vi "数据查询_仪器日志.vi"() -> ()   [LabVIEW 2016, in "数据查询.lvlib"]
uses:
  <vilib>/Utility/miscctls.llb/LVPointTypeDef.ctl
  <vilib>/Utility/miscctls.llb/LVRowAndColumnUnsignedTypeDef.ctl
  <userlib>/_OpenG.lib/array/array.llb/Sort 2D Array (String)__ogtk.vi
  <userlib>/_LVST/sqlite_api/Core/Tables/SQLite_List Columns.vi
  <vilib>/addons/database/_DB Variant To Data/Database Variant To Data.xnode
panel:
  out "布尔":bool=TRUE
  in  "列表框":i32(listbox)
  in  "页":i32 format="第%.0f页"
  in  "每页条数":i32=1000
  in  "向后按钮":bool
  in  "向前按钮":bool
  in  "导出":bool
  in  "查询":bool
  out "数据表":string[][](table)
  in  "结束日期":string="2050/01/01"
  in  "起始日期":string="2010/01/01"
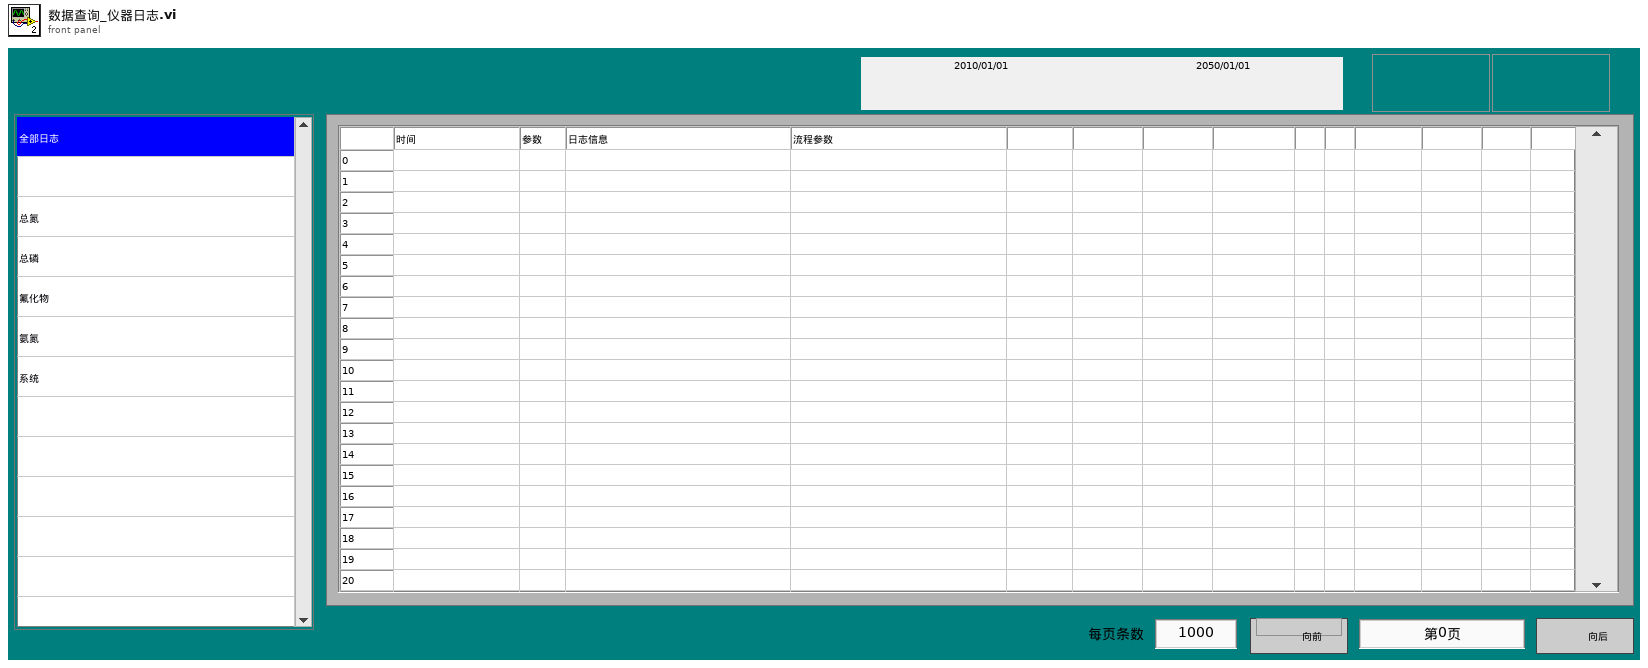
[diagram p1: front panel]
types:
  T1 = typedef "LVPointTypeDef.ctl" = cluster{"Horizontal":i16, "Vertical":i16}
  T2 = typedef "LVDateTimeRec.ctl" = cluster{"秒数的小数部分":dbl, "秒":i32, "分":i32, "时":i32, "日":i32, "月":i32, "年":i32, "天数（周）":i32, "天数（年）":i32, "DST":i32}
  T3 = typedef "Rendezvous RefNum" = refnum<k1>
  T4 = typedef "数据查询.lvlib/数据查询单选控件.ctl" = enum32{"数据查询", "仪器数据", "仪器日志", "报警信息", "校准日志"}
  T5 = typedef "数据库类型.ctl" = enum16{"Access", "SQLite"}
  T6 = enum8{"Enabled", "Disabled", "Disabled and Grayed Out"}
  T7 = typedef "LVRowAndColumnUnsignedTypeDef.ctl" = cluster{"Row":u32, "Column":u32}
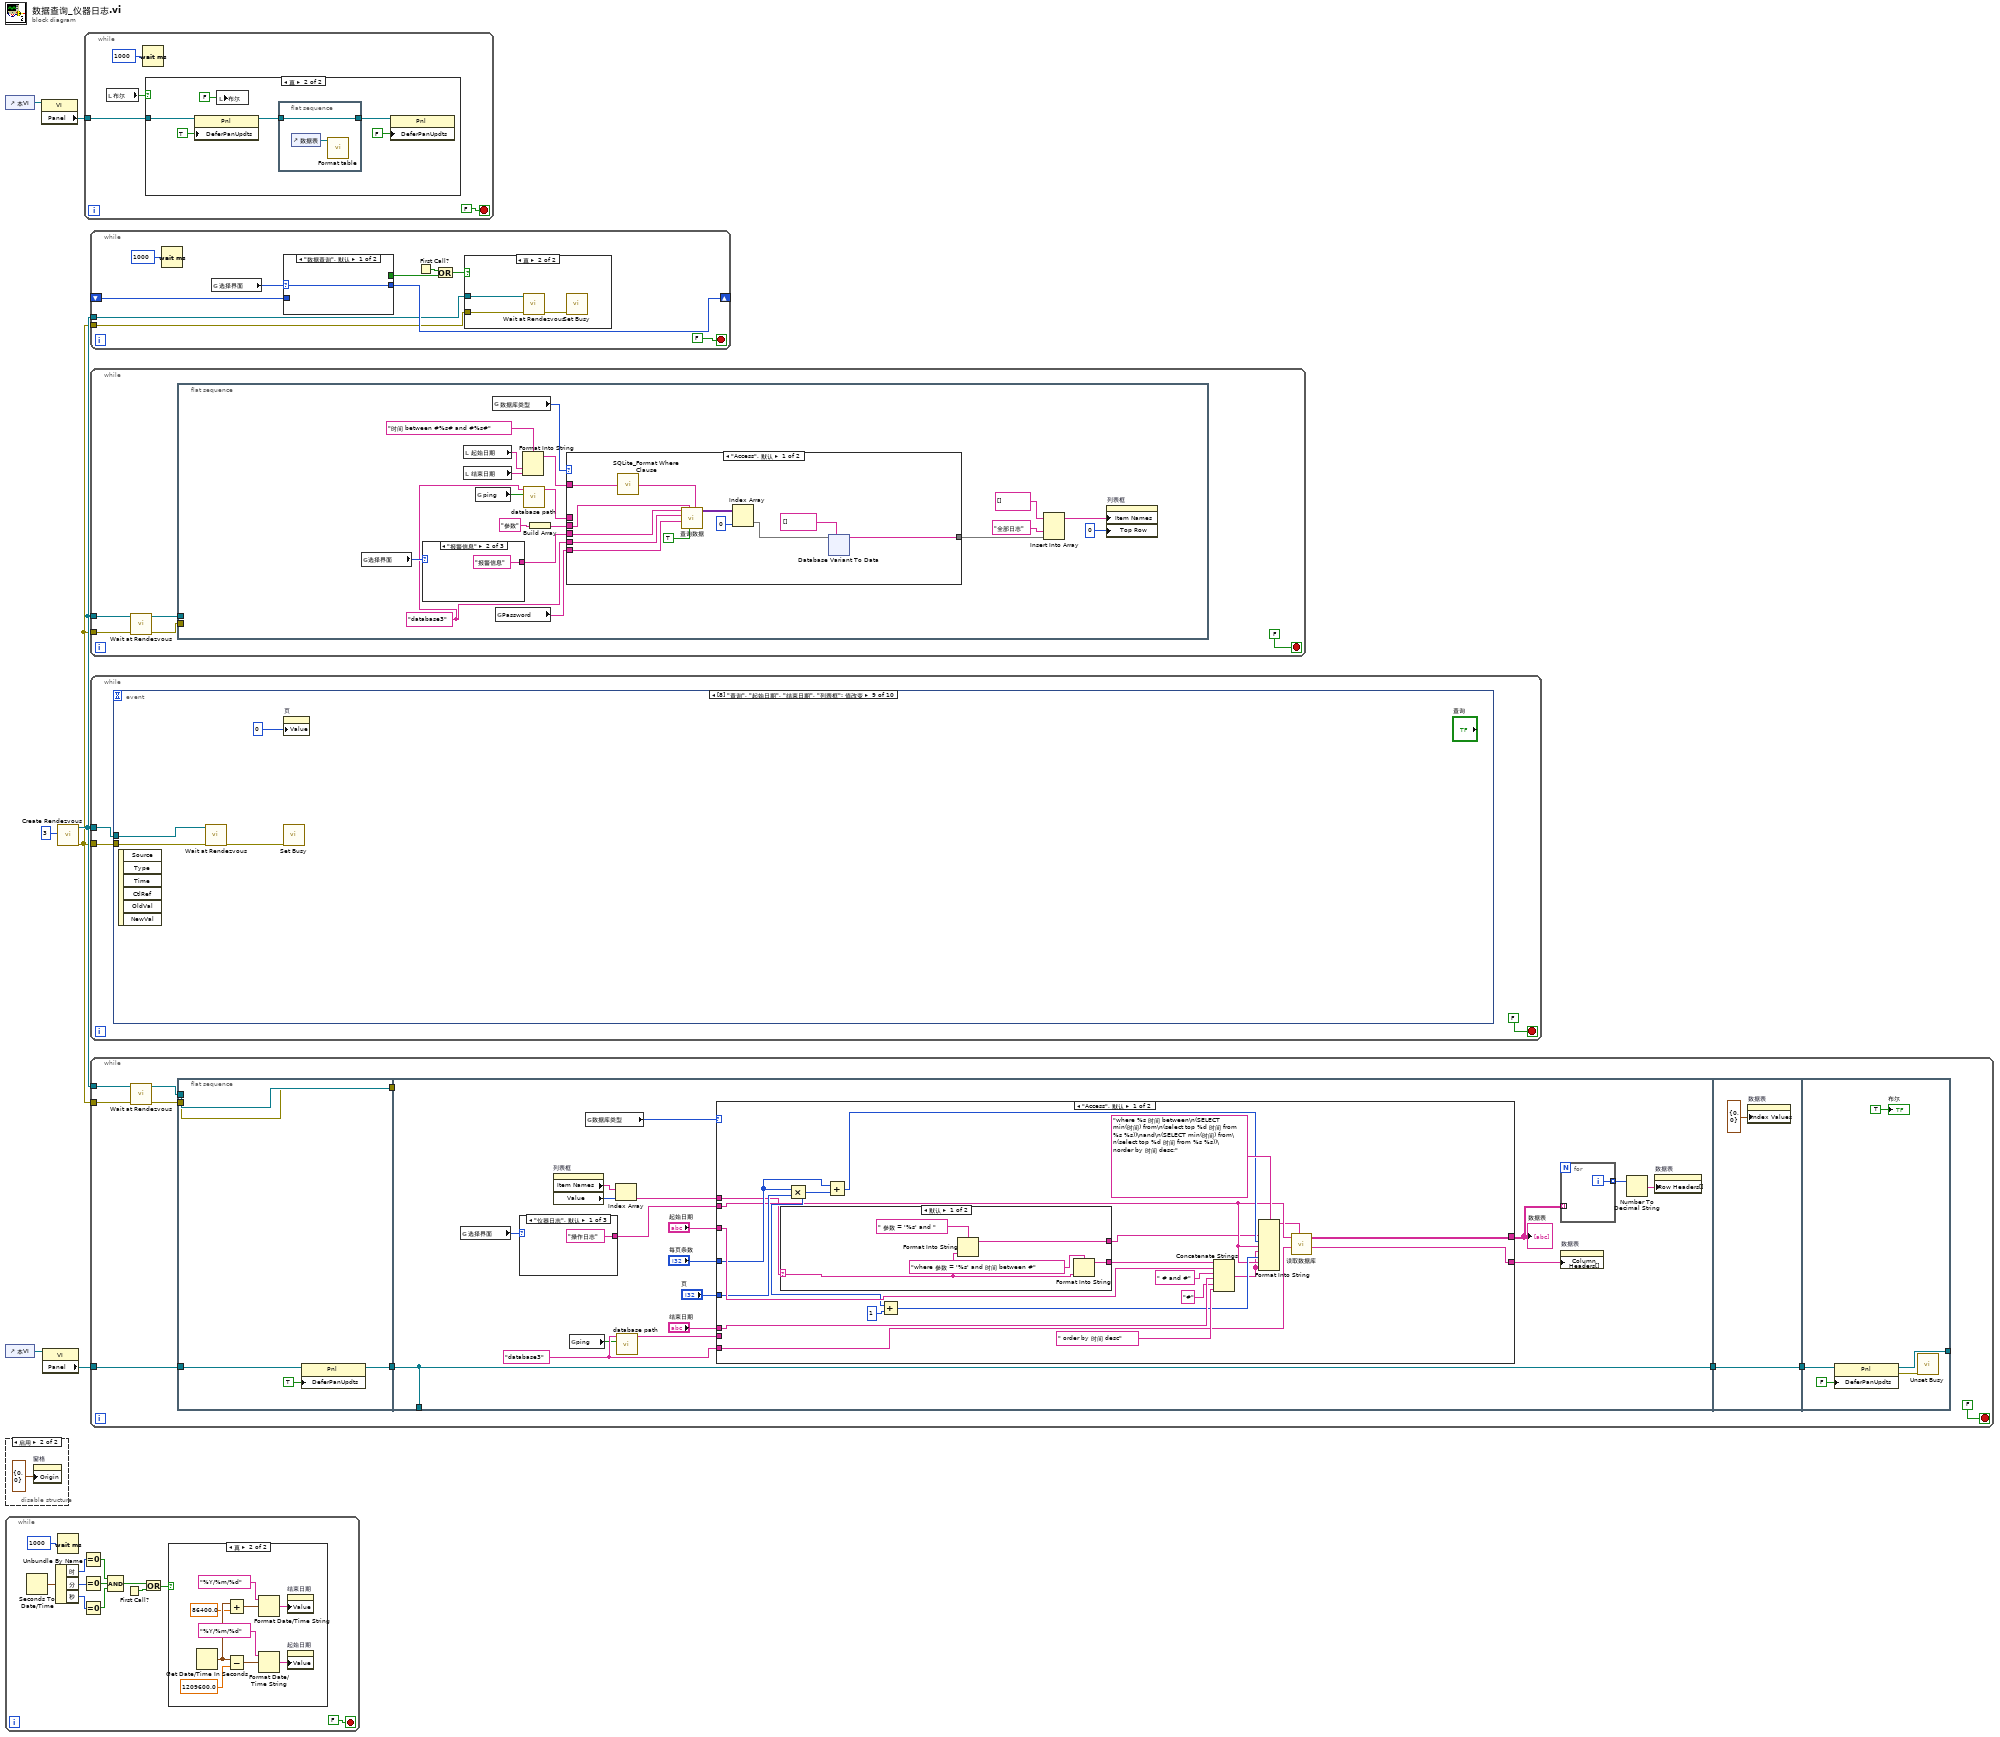
[diagram p0: block diagram]
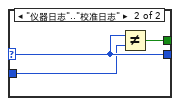
[diagram p4: hidden frame]
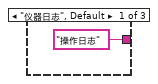
[diagram p5: hidden frame]
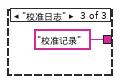
[diagram p6: hidden frame]
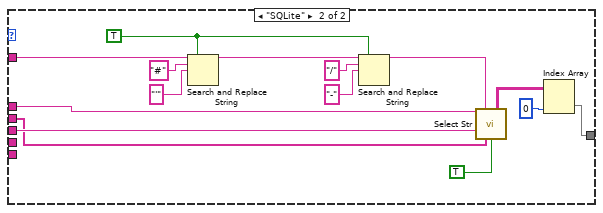
[diagram p7: hidden frame]
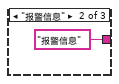
[diagram p8: hidden frame]
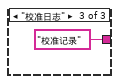
[diagram p9: hidden frame]
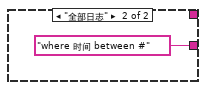
[diagram p10: hidden frame]
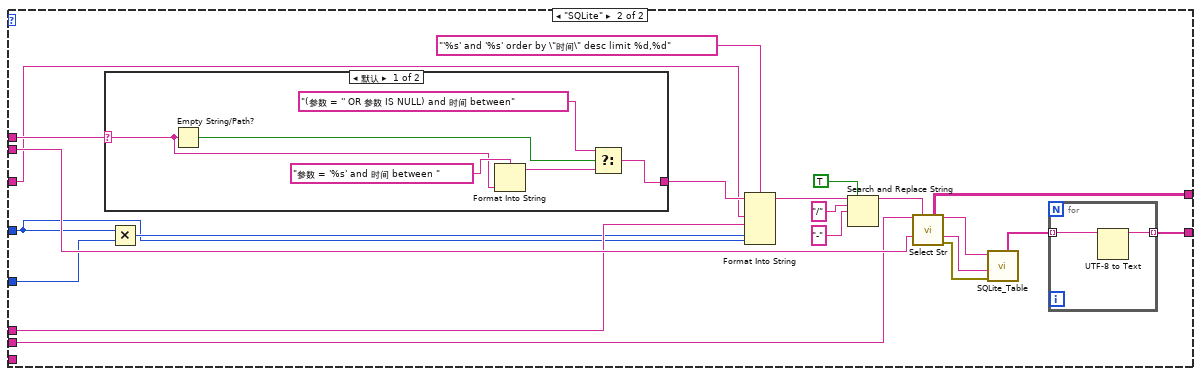
[diagram p11: hidden frame]
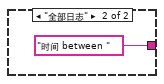
[diagram p12: hidden frame]
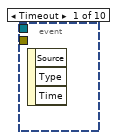
[diagram p14: hidden frame]
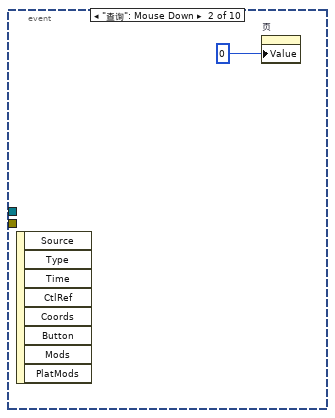
[diagram p15: hidden frame]
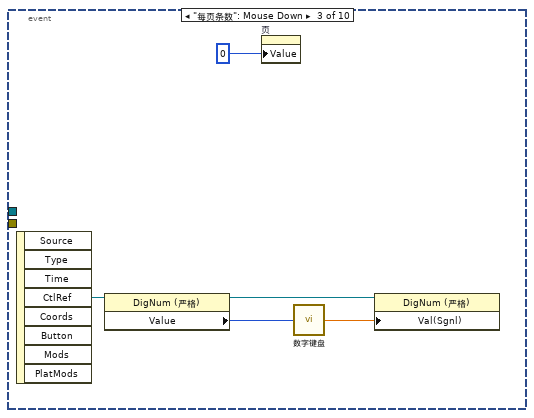
[diagram p16: hidden frame]
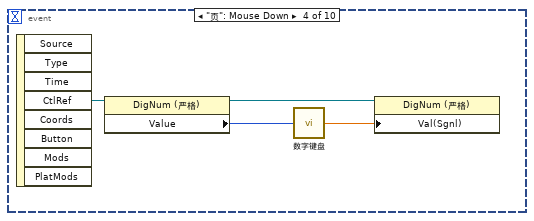
[diagram p17: hidden frame]
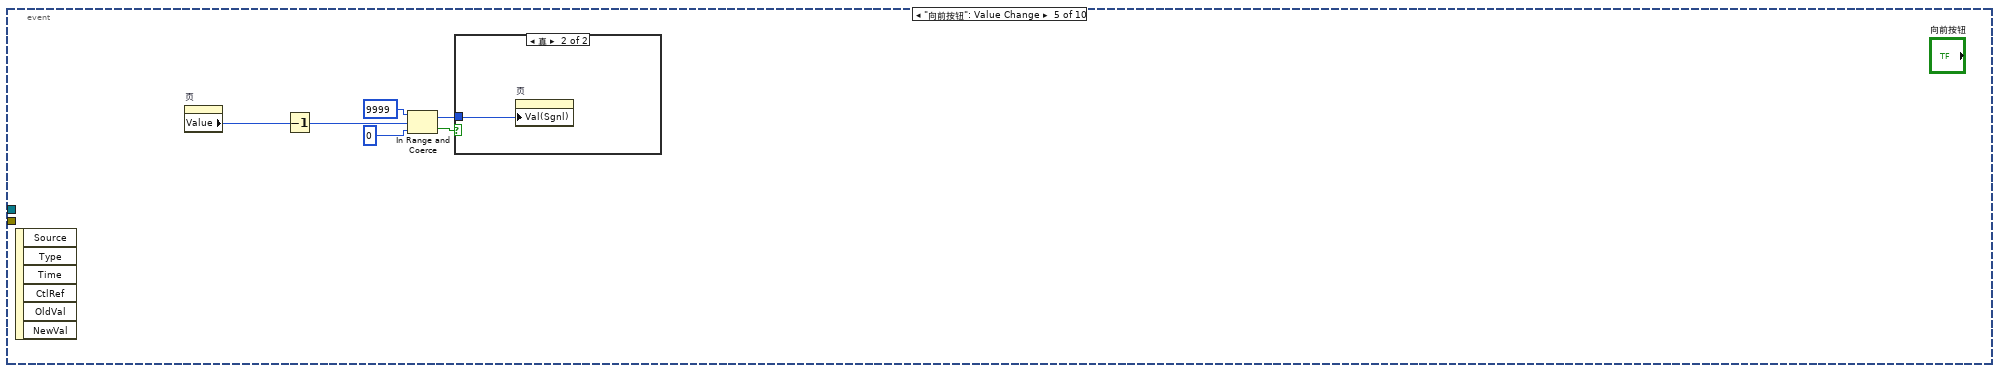
[diagram p18: hidden frame]
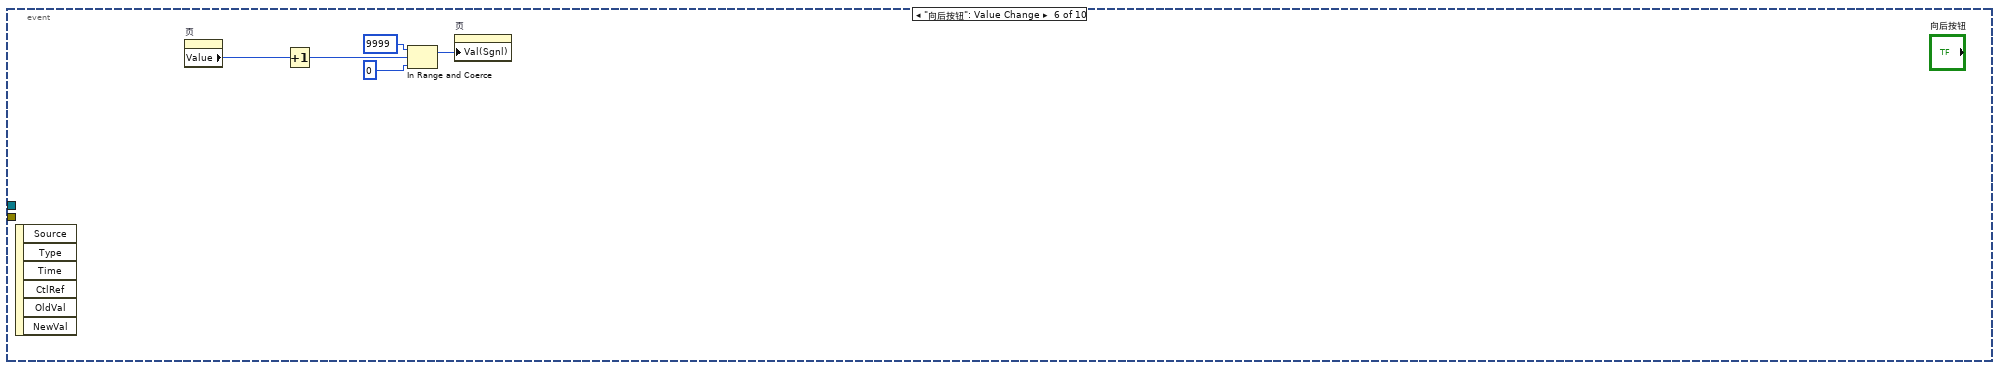
[diagram p20: hidden frame]
diagram:
  n1 = control-ref of="本VI"() -> (w2:refnum<vi>)
  n2 = control-ref of="本VI"() -> (w6:refnum<vi>)
  n3 = disable-structure shown="启用" {
    frame Disabled {
    }
    frame Enabled {
      n4 = property on="窗格" class="Pane"("Origin"=T1 {"Horizontal"=0, "Vertical"=0} ("原点")) -> ()  [unwired: 2 in, 2 out]
    }
  }
  n5 = while {
    stop <- FALSE stop-if-true
    n6 = Seconds To Date/Time() -> (date time rec=w20:T2)  [unwired: 2 in]
    n7 = Unbundle By Name(w20) -> ("时"=w19:i32, "分"=w18:i32, "秒"=w17:i32)
    n8 = Wait (ms)(milliseconds to wait=u32 1000 ("等待时间（毫秒）")) -> ()  [unwired: 1 out]
    n9 = Equal To 0?(x=w19) -> (x = 0?=w16:bool)
    n10 = Equal To 0?(x=w18) -> (x = 0?=w15:bool)
    n11 = Equal To 0?(x=w17) -> (x = 0?=w14:bool)
    n12 = Compound Arithmetic op=AND ("复合运算")(w16, w15, w14) -> (w11:bool)
    n13 = First Call?() -> (First Call?: T/F=w10:bool)
    n14 = Or(x=w11, y=w10) -> (x .or. y?=w9:bool)
    n15 = case shown="真" w9 {
      frame False {
      }
      frame True {
        n16 = Get Date/Time In Seconds() -> (seconds since 1Jan1904=w25:timestamp)
        n17 = Add(x=w25, y=86400.0) -> (x+y=w23:timestamp)
        n18 = Subtract(x=w25, y=1209600.0) -> (x-y=w26:timestamp)
        n19 = Format Date/Time String(time format string (%c)="%Y/%m/%d" ("时间格式字符串(%c)"), seconds (now)=w23) -> (date/time string=w22:string)  [unwired: 1 in]
        n20 = Format Date/Time String(time format string (%c)="%Y/%m/%d" ("时间格式字符串(%c)"), seconds (now)=w26) -> (date/time string=w28:string)  [unwired: 1 in]
        n21 = property on="结束日期" class="Str"("Value"=w22) -> ()  [unwired: 2 in, 2 out]
        n22 = property on="起始日期" class="Str"("Value"=w28) -> ()  [unwired: 2 in, 2 out]
      }
    }
  }
  n23 = property class="VI"(reference=w2) -> ("Panel"=w1:refnum<vi>)  [unwired: 1 in, 2 out]
  n24 = property class="VI"(reference=w6) -> ("Panel"=w5:refnum<vi>)  [unwired: 1 in, 2 out]
  n25 = call <vilib>:"Create Rendezvous.vi"("size (2)"=3) -> ("error out"=w3:errorcluster, "rendezvous"=w4:T3)  [unwired: 4 in, 1 out]
  n26 = while {
    tunnel: w1 -> [w32]
    stop <- FALSE stop-if-true
    n27 = local read "布尔"() -> (w31:bool)
    n28 = Wait (ms)(milliseconds to wait=u32 1000 ("等待时间（毫秒）")) -> ()  [unwired: 1 out]
    n29 = case shown="真" w31 {
      tunnel: w32 -> [_ w38]
      frame False {
      }
      frame True {
        n30 = property class="Pnl"(reference=w38, "DeferPanUpdts"=TRUE ("延迟前面板更新")) -> (reference out=w37:refnum<vi>)  [unwired: 1 in, 1 out]
        n31 = local write "布尔"(FALSE ("布尔")) -> ()
        n32 = flat-sequence {
          tunnel: [w40] -> w36
          tunnel: w37 -> [w40]
          frame #0 {
            n33 = control-ref of="数据表"() -> (w41:refnum<vi>)
            n34 = call "Format table.vi"("Table输入"=w41) -> ()  [unwired: 11 in]
          }
        }
        n35 = property class="Pnl"(reference=w36, "DeferPanUpdts"=FALSE ("延迟前面板更新")) -> ()  [unwired: 1 in, 2 out]
      }
    }
  }
  n36 = while {
    shift-right: [w48] -> _
    shift-left: _ -> [w47]
    tunnel: w4 -> [w45]
    tunnel: w3 -> [w42]
    stop <- FALSE stop-if-true
    n37 = Wait (ms)(milliseconds to wait=u32 1000 ("等待时间（毫秒）")) -> ()  [unwired: 1 out]
    n38 = global read "全局变量.vi" "选择界面"() -> (w49:T4)
    n39 = case shown="\"数据查询\", 默认" w49 {
      selector: w49 -> [w55 w58]
      tunnel: [w55 w58] -> w48
      tunnel: w47 -> [_ w57]
      tunnel: [_ w56] -> w46
      frame "数据查询", Default {
      }
      frame "仪器日志".."校准日志" {
        n40 = Not Equal?(x=w58, y=w57) -> (x != y?=w56:bool)
      }
    }
    n41 = First Call?() -> (First Call?: T/F=w43:bool)
    n42 = Or(x=w43, y=w46) -> (x .or. y?=w44:bool)
    n43 = case shown="真" w44 {
      tunnel: w45 -> [_ w54]
      tunnel: w42 -> [_ w53]
      frame False {
      }
      frame True {
        n44 = call <vilib>:"Wait at Rendezvous.vi"("error in (no error)"=w53, "rendezvous"=w54) -> ("error out"=w52:errorcluster)  [unwired: 3 in, 2 out]
        n45 = call <vilib>:"Set Busy.vi"("error in (no error)"=w52) -> ()  [unwired: 9 in, 2 out]
      }
    }
  }
  n46 = while {
    tunnel: w4 -> [w62]
    tunnel: w3 -> [w61]
    stop <- FALSE stop-if-true
    n47 = call <vilib>:"Wait at Rendezvous.vi"("error in (no error)"=w61, "rendezvous"=w62) -> ("error out"=w59:errorcluster, "rendezvous out"=w60:T3)  [unwired: 3 in, 1 out]
    n48 = flat-sequence {
      tunnel: w60 -> [_]
      tunnel: w59 -> [_]
      frame #0 {
        w68 = "database3" ("database")
        n49 = global read "全局变量.vi" "选择界面"() -> (w71:T4)
        n50 = case shown="\"报警信息\"" w71 {
          tunnel: ["操作日志" "报警信息" "校准记录"] -> w70
          frame "仪器日志", Default {
          }
          frame "报警信息" {
          }
          frame "校准日志" {
          }
        }
        n51 = local read "起始日期"() -> (w77:string)
        n52 = local read "结束日期"() -> (w76:string)
        n53 = global read "全局变量.vi" "ping"() -> (w67:bool)
        n54 = global read "外部调用接口全局变量.vi" "数据库类型"() -> (w65:T5)
        n55 = global read "外部调用接口全局变量.vi" "Password"() -> (w64:string)
        n56 = Format Into String(format string="时间 between #%s# and #%s#" ("格式字符串"), w77, w76) -> (resulting string=w73:string)  [unwired: 2 in, 1 out]
        n57 = call "database path.vi"("ping"=w67, "database"=w68) -> ("Path out"=w69:string)  [unwired: 8 in, 1 out]
        n58 = Build Array("参数") -> (w72:string[])
        n59 = case shown="\"Access\", 默认" w65 {
          tunnel: w70 -> [w96 w149]
          tunnel: w72 -> [w95 w148]
          tunnel: [w89 w135] -> w66
          tunnel: w73 -> [w88 w144]
          tunnel: w68 -> [w86 _]
          tunnel: w69 -> [_ w136]
          tunnel: w64 -> [w85 _]
          frame "Access", Default {
            n60 = call <userlib>:"SQLite_Format Where Clause.vi"("Where clause"=w88) -> ("String"=w87:string)  [unwired: 4 in]
            n61 = call "查询数据.vi"("condition"=w87, "Distinct"=TRUE, "columns"=w95, "Password"=w85, "database"=w86, "table"=w96) -> ("data"=w94:variant[][])  [unwired: 4 in, 1 out]
            n62 = Index Array(array=w94, index (col)=0 ("禁用的索引 (列)")) -> (element=w93:variant[])  [unwired: 1 in]
            n63 = xnode "Database Variant To Data"("database variant"=w93, "type"=string[] []) -> ("data"=w89:string[])  [unwired: 1 in, 1 out]
          }
          frame "SQLite" {
            w137 = TRUE ("替换全部？(F)")
            n64 = Search and Replace String(replace all?=w137, input string=w144, search string="#" ("搜索字符串"), replace string="'" ("替换字符串(\"\")")) -> (result string=w139:string)  [unwired: 4 in, 3 out]
            n65 = Search and Replace String(replace all?=w137, input string=w139, search string="/" ("搜索字符串"), replace string="-" ("替换字符串(\"\")")) -> (result string=w138:string)  [unwired: 4 in, 3 out]
            n66 = call "Select Str.vi"("DB Path"=w136, "Where Clause"=w138, "Tables Name"=w149, "Columns"=w148, "Distinct"=TRUE) -> ("Results"=w146:string[][])  [unwired: 7 in, 3 out]
            n67 = Index Array(array=w146, index (col)=0 ("禁用的索引 (列)")) -> (element=w135:string[])  [unwired: 1 in]
          }
        }
        n68 = Insert Into Array(array=string[] [], new element #1="全部日志" ("新元素/子数组"), new element #2=w66) -> (w75:string[])  [unwired: 1 in]
        n69 = property on="列表框" class="LstBox (严格)"("Item Names"=w75, "Top Row"=0 ("顶行")) -> ()  [unwired: 2 in, 2 out]
      }
    }
  }
  n70 = while {
    tunnel: w4 -> [w151]
    tunnel: w3 -> [w150]
    stop <- FALSE stop-if-true
    n71 = event shown="[8] \"查询\", \"起始日期\", \"结束日期\", \"列表框\": 值改变" {
      selector: _ -> [_ _ _ _ _ _ _ _ _ _]
      dyn-events: _ -> [_ _ _ _ _ _ _ _ _ _]
      timeout: _ -> [_ _ _ _ _ _ _ _ _ _]
      tunnel: w151 -> [_ _ _ _ _ _ _ _ w221 w225]
      tunnel: w150 -> [_ _ _ _ _ _ _ _ w220 w224]
      event Timeout {
        n72 = event-data() -> ()  [unwired: 1 in, 3 out]
      }
      event "查询": Mouse Down {
        n73 = event-data() -> ()  [unwired: 1 in, 8 out]
        n74 = property on="页" class="DigNum (严格)"("Value"=0 ("页")) -> ()  [unwired: 2 in, 2 out]
      }
      event "每页条数": Mouse Down {
        n75 = event-data() -> ("CtlRef"=w158:refnum<vi>)  [unwired: 1 in, 7 out]
        n76 = property class="DigNum (严格)"(reference=w158) -> (reference out=w155:refnum<vi>, "Value"=w157:i32)  [unwired: 1 in, 1 out]
        n77 = property on="页" class="DigNum (严格)"("Value"=0 ("页")) -> ()  [unwired: 2 in, 2 out]
        n78 = call "数字键盘.vi"("OldNumber"=w157) -> ("NewNumber"=w156:sgl)
        n79 = property class="DigNum (严格)"(reference=w155, "Val(Sgnl)"=w156) -> ()  [unwired: 1 in, 2 out]
      }
      event "页": Mouse Down {
        n80 = event-data() -> ("CtlRef"=w162:refnum<vi>)  [unwired: 1 in, 7 out]
        n81 = property class="DigNum (严格)"(reference=w162) -> (reference out=w159:refnum<vi>, "Value"=w161:i32)  [unwired: 1 in, 1 out]
        n82 = call "数字键盘.vi"("OldNumber"=w161) -> ("NewNumber"=w160:sgl)
        n83 = property class="DigNum (严格)"(reference=w159, "Val(Sgnl)"=w160) -> ()  [unwired: 1 in, 2 out]
      }
      event "向前按钮": Value Change {
        n84 = event-data() -> ()  [unwired: 1 in, 6 out]
        n85 = property on="页" class="DigNum (严格)"() -> ("Value"=w168:i32)  [unwired: 2 in, 2 out]
        n86 = Decrement(x=w168) -> (x-1=w167:i32)
        n87 = In Range and Coerce(upper limit=9999 ("上限"), x=w167, lower limit=0 ("下限")) -> (coerced(x)=w164:i32, In Range?=w163:bool)
        n88 = case shown="真" w163 {
          tunnel: w164 -> [_ w169]
          frame False {
          }
          frame True {
            n89 = property on="页" class="DigNum (严格)"("Val(Sgnl)"=w169) -> ()  [unwired: 2 in, 2 out]
          }
        }
      }
      event "向后按钮": Value Change {
        n90 = event-data() -> ()  [unwired: 1 in, 6 out]
        n91 = property on="页" class="DigNum (严格)"() -> ("Value"=w174:i32)  [unwired: 2 in, 2 out]
        n92 = Increment(x=w174) -> (x+1=w173:i32)
        n93 = In Range and Coerce(upper limit=u32 9999 ("上限"), x=w173, lower limit=u32 0 ("下限")) -> (coerced(x)=w170:u32)  [unwired: 1 out]
        n94 = property on="页" class="DigNum (严格)"("Val(Sgnl)"=w170) -> ()  [unwired: 2 in, 2 out]
      }
      event "导出": Value Change {
        n95 = event-data() -> ("CtlRef"=w175:refnum<vi>)  [unwired: 1 in, 5 out]
        n96 = property class="Bool"(reference=w175, "DisabledEnum"=T6."Disabled and Grayed Out" ("禁用")) -> (reference out=w179:refnum<vi>, error out=w180:errorcluster)  [unwired: 1 in]
        n97 = flat-sequence {
          tunnel: w180 -> [_]
          tunnel: [w199] -> w178
          tunnel: w179 -> [w199]
          tunnel: "导出" -> [_]
          frame #0 {
            n98 = local read "数据表"() -> (w203:string[][])
            n99 = call-poly <userlib>:"Sort Array__ogtk.vi"("Column/Row to Sort By"=u32 0, "Sort By in"=enum16{"row", "column"}."column", "Order"=enum16{"ascending", "descending"}."ascending", "Array in"=w203) -> ("Sorted Array out"=w185:string[][])  [unwired: 4 in, 3 out]
            n100 = for {
              tunnel: w185 -> [w212] mode=indexing
              tunnel: [w211] -> w189 mode=indexing
              i -> [w213]
              n101 = Increment(x=w213) -> (x+1=w209:i32)
              n102 = Number To Decimal String(number=w209) -> (decimal integer string=w208:string)  [unwired: 1 in]
              n103 = Insert Into Array(array=w212, index=0 ("索引"), new element=w208) -> (w211:string[])
            }
            n104 = property on="数据表" class="Tbl (严格)"() -> ("Column Headers[]"=w192:string[])  [unwired: 2 in, 2 out]
            n105 = property on="列表框" class="LstBox (严格)"() -> ("Item Names"=w184:string[], "Value"=w183:i32)  [unwired: 2 in, 2 out]
            n106 = Insert Into Array(array=w192, index=0 ("索引"), new element="序号" ("新元素/子数组")) -> (w193:string[])
            n107 = Index Array(array=w184, index=w183) -> (element=w182:string)
            n108 = Format Date/Time String(time format string (%c)="%y_%m_%d" ("时间格式字符串(%c)")) -> (date/time string=w196:string)  [unwired: 2 in]
            n109 = Concatenate Strings(w182, "_" ("字符串"), w196) -> (w194:string)
            n110 = Insert Into Array(array=string[][] [], new element #1=w193, new element #2=w189) -> (w188:string[][])  [unwired: 2 in]
            n111 = call "数据导出Excel.vi"("text data"=w188, "default name"=w194) -> ("error out"=w187:errorcluster, "布尔"=w186:bool)  [unwired: 8 in]
            n112 = case shown="真" w186 {
              tunnel: w187 -> [_ w205]
              frame False {
              }
              frame True {
                n113 = case shown="错误" w205 {
                  tunnel: ["导出成功" ("消息") "导出失败" ("消息")] -> w204
                  frame No Error {
                  }
                  frame Error {
                  }
                }
                n114 = One Button Dialog(message=w204) -> ()  [unwired: 1 in, 1 out]
              }
            }
          }
        }
        n115 = property class="Bool"(reference=w178, "DisabledEnum"=T6."Enabled" ("禁用")) -> ()  [unwired: 1 in, 2 out]
      }
      event "起始日期", "结束日期": Mouse Down {
        n116 = event-data() -> ("CtlRef"=w218:refnum<vi>)  [unwired: 1 in, 7 out]
        n117 = property class="Str"(reference=w218) -> (reference out=w216:refnum<vi>, "Value"=w217:string)  [unwired: 1 in, 1 out]
        n118 = property on="页" class="DigNum (严格)"("Value"=0 ("页")) -> ()  [unwired: 2 in, 2 out]
        n119 = call "日期键盘.vi"("原值"=w217) -> ("x+y"=w215:string)  [unwired: 10 in]
        n120 = property class="Str"(reference=w216, "Val(Sgnl)"=w215) -> ()  [unwired: 1 in, 2 out]
      }
      event "查询", "起始日期", "结束日期", "列表框": Value Change {
        n121 = event-data() -> ()  [unwired: 1 in, 6 out]
        n122 = call <vilib>:"Wait at Rendezvous.vi"("error in (no error)"=w220, "rendezvous"=w221) -> ("error out"=w219:errorcluster)  [unwired: 3 in, 2 out]
        n123 = property on="页" class="DigNum (严格)"("Value"=0 ("页")) -> ()  [unwired: 2 in, 2 out]
        n124 = call <vilib>:"Set Busy.vi"("error in (no error)"=w219) -> ()  [unwired: 9 in, 2 out]
      }
      event "页", "每页条数": Value Change {
        n125 = event-data() -> ()  [unwired: 1 in, 6 out]
        n126 = call <vilib>:"Wait at Rendezvous.vi"("error in (no error)"=w224, "rendezvous"=w225) -> ("error out"=w223:errorcluster)  [unwired: 3 in, 2 out]
        n127 = call <vilib>:"Set Busy.vi"("error in (no error)"=w223) -> ()  [unwired: 9 in, 2 out]
      }
    }
  }
  n128 = while {
    tunnel: w4 -> [w235]
    tunnel: w3 -> [w234]
    tunnel: w5 -> [w229]
    stop <- FALSE stop-if-true
    n129 = call <vilib>:"Wait at Rendezvous.vi"("error in (no error)"=w234, "rendezvous"=w235) -> ("error out"=w232:errorcluster, "rendezvous out"=w233:T3)  [unwired: 3 in, 1 out]
    n130 = flat-sequence {
      tunnel: w232 -> [w240]
      tunnel: w233 -> [w241]
      tunnel: [w241] -> w231
      tunnel: [w240] -> w230
      tunnel: w229 -> [w239]
      tunnel: [w237] -> w228
      tunnel: w231 -> [_]
      tunnel: w230 -> [_]
      tunnel: [w242] -> _
      tunnel: w228 -> [w242]
      tunnel: [w242] -> w227
      tunnel: w227 -> [w321]
      tunnel: [w321] -> w226
      tunnel: [w326] -> _
      tunnel: w226 -> [w327]
      frame #0 {
        n131 = property class="Pnl"(reference=w239, "DeferPanUpdts"=TRUE ("延迟前面板更新")) -> (reference out=w237:refnum<vi>)  [unwired: 1 in, 1 out]
      }
      frame #1 {
        w245 = "database3" ("database")
        n132 = global read "全局变量.vi" "选择界面"() -> (w248:T4)
        n133 = case shown="\"仪器日志\", 默认" w248 {
          tunnel: ["操作日志" "报警信息" "校准记录"] -> w247
          frame "仪器日志", Default {
          }
          frame "报警信息" {
          }
          frame "校准日志" {
          }
        }
        n134 = property on="列表框" class="LstBox (严格)"() -> ("Item Names"=w256:string[], "Value"=w257:i32)  [unwired: 2 in, 2 out]
        n135 = global read "全局变量.vi" "ping"() -> (w244:bool)
        n136 = global read "外部调用接口全局变量.vi" "数据库类型"() -> (w243:T5)
        n137 = Index Array(array=w256, index=w257) -> (element=w253:string)
        n138 = call "database path.vi"("ping"=w244, "database"=w245) -> ("Path out"=w246:string)  [unwired: 8 in, 1 out]
        n139 = case shown="\"Access\", 默认" w243 {
          tunnel: "起始日期" -> [w283 w302]
          tunnel: "结束日期" -> [w282 w301]
          tunnel: [w279 w291] -> w255
          tunnel: [w277 w306] -> w254
          tunnel: "每页条数" -> [w271 w293]
          tunnel: "页" -> [w270 w295]
          tunnel: w247 -> [w269 w310]
          tunnel: w245 -> [w267 _]
          tunnel: w253 -> [w265 w305]
          tunnel: w246 -> [_ w290]
          frame "Access", Default {
            n140 = case shown="默认" w265 {
              selector: w265 -> [w285 _]
              tunnel: [w288 "where 时间 between #" ("condition")] -> w263
              tunnel: [w284 _] -> w264
              frame Default {
                n141 = Format Into String(format string=" 参数 = '%s' and " ("condition"), w285) -> (resulting string=w284:string)  [unwired: 2 in, 1 out]
                n142 = Format Into String(format string="where 参数 = '%s' and 时间 between #" ("condition"), w285) -> (resulting string=w288:string)  [unwired: 2 in, 1 out]
              }
              frame "全部日志" {
              }
            }
            n143 = Multiply(x=w271, y=w270) -> (x*y=w275:i32)
            n144 = Add(x=w271, y=w275) -> (x+y=w273:i32)
            n145 = Add(x=w275, y=u32 1) -> (x+y=w272:u32)
            n146 = Concatenate Strings(w263, w283, " # and #" ("condition"), w282, "#" ("condition"), " order by 时间 desc" ("字符串")) -> (w268:string)
            n147 = Format Into String(format string="where %s 时间 between\n(SELECT min(时间) from\n(select top %d 时间 from %s %s))\nand\n(SELECT min(时间) from\n(select top %d 时间 from %s %s))\norder by 时间 desc;" ("格式字符串"), w264, w273, w269, w268, w272, w269, w268) -> (resulting string=w266:string)  [unwired: 2 in, 1 out]
            n148 = call "读取数据库.vi"("condition"=w266, "database"=w267, "组合框"=w269) -> ("columns"=w279:string[], "表格"=w277:string[][])  [unwired: 5 in, 2 out]
          }
          frame "SQLite" {
            n149 = case shown="默认" w305 {
              selector: w305 -> [w313 _]
              tunnel: [w314 "时间 between " ("condition")] -> w304
              frame Default {
                n150 = Empty String/Path?(string/path=w313) -> (empty?=w318:bool)
                n151 = Format Into String(format string="参数 = '%s' and 时间 between " ("condition"), w313) -> (resulting string=w315:string)  [unwired: 2 in, 1 out]
                n152 = Select(t="(参数 = '' OR 参数 IS NULL) and 时间 between" ("condition"), s=w318, f=w315) -> (s? t:f=w314:string)
              }
              frame "全部日志" {
              }
            }
            n153 = Multiply(x=w293, y=w295) -> (x*y=w294:i32)
            n154 = Format Into String(format string="'%s' and '%s' order by \"时间\" desc limit %d,%d" ("格式字符串"), initial string=w304, w302, w301, w294, w293) -> (resulting string=w298:string)  [unwired: 1 in, 1 out]
            n155 = Search and Replace String(replace all?=TRUE ("替换全部？(F)"), input string=w298, search string="/" ("搜索字符串"), replace string="-" ("替换字符串(\"\")")) -> (result string=w297:string)  [unwired: 4 in, 3 out]
            n156 = call "Select Str.vi"("DB Path"=w290, "Where Clause"=w297, "Tables Name"=w310) -> ("Results"=w306:string[][], "DB Path Out"=w309:string, "Table Name Out"=w308:string, "error out"=w307:errorcluster)  [unwired: 9 in]
            n157 = call-poly <userlib>:"SQLite_Table.vi"("DB Path"=w309, "Table Name"=w308, "error in (no error)"=w307) -> ("Columns"=w292:string[])  [unwired: 4 in, 3 out]
            n158 = for {
              tunnel: w292 -> [w312] mode=indexing
              tunnel: [w311] -> w291 mode=indexing
              n159 = UTF-8 to Text(11:w312) -> (3:w311:string)  [unwired: 2 in, 1 out]
            }
          }
        }
        "数据表" <- w254
        n160 = for {
          tunnel: [w320] -> w259 mode=indexing
          tunnel: w254 -> [_] mode=indexing
          i -> [w320]
        }
        n161 = property on="数据表" class="Tbl (严格)"("Column Headers[]"=w255) -> ()  [unwired: 2 in, 2 out]
        n162 = Number To Decimal String(number=w259) -> (decimal integer string=w258:string[])  [unwired: 1 in]
        n163 = property on="数据表" class="Tbl (严格)"("Row Headers[]"=w258) -> ()  [unwired: 2 in, 2 out]
      }
      frame #2 {
        n164 = property on="数据表" class="Tbl (严格)"("Index Values"=T7 {"Row"=0, "Column"=0} ("索引值")) -> ()  [unwired: 2 in, 2 out]
      }
      frame #3 {
        n165 = property class="Pnl"(reference=w327, "DeferPanUpdts"=FALSE ("延迟前面板更新")) -> (reference out=w326:refnum<vi>, error out=w324:errorcluster)  [unwired: 1 in]
        n166 = call <vilib>:"Unset Busy.vi"("error in (no error)"=w324) -> ()  [unwired: 10 in, 1 out]
        "布尔" <- TRUE
      }
    }
  }
